vi "MsgLog.vi"(10 "OP_ID":refnum<vi>) -> ()   [LabVIEW 2019, in "MsgShowAndLog.lvlib"]
uses:
  MsgShowAndLog.lvlib
  Ctrl/MsgPageSelect.ctl
  Ctrl/MsgTyp.ctl
  Ctrl/MsgDataInput.ctl
  Ctrl/LogType.ctl
  <vilib>/Utility/miscctls.llb/LVPositionTypeDef.ctl
  global/MsgQue.vi
  Commonly VI.lvlib
panel:
  in  "OP":string
  in  "DataIn":T1={"MsgPageSelect"=enum."Action", "LogType"=enum."Manual", "Msg"="", "Time"=""}
  in  "Type":T4=enum."IO"
  in  "Enum":T2
  in  "error in":errorcluster
  in  "Main_msgTable":enum32{"系統訊息", "通訊訊息", "IO訊息", "動作訊息", "報警訊息"}(tab)
  in  "SystemMsg":i32(listbox)
  in  "RobotMsg":i32(listbox)
  in  "IOMsg":i32(listbox)
  in  "ActionMsg":i32(listbox)
  in  "AlarmMsg":i32(listbox)
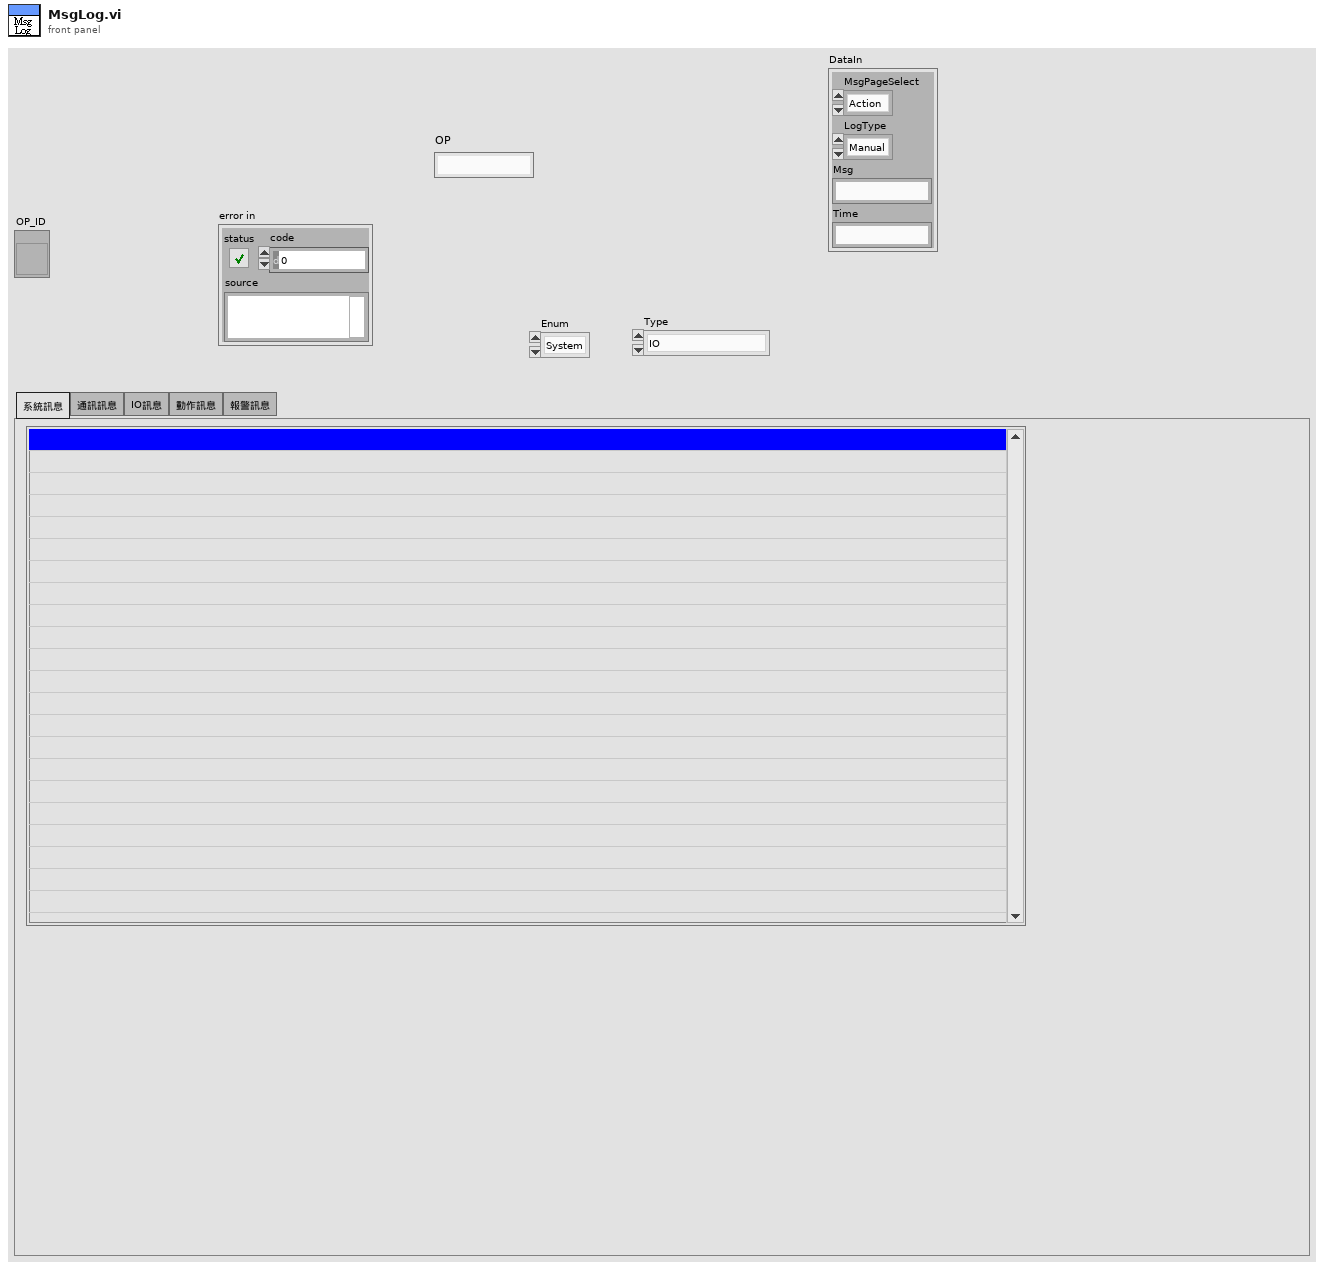
[diagram p1: front panel]
types:
  T1 = typedef "MsgDataInput.ctl" = cluster{"MsgPageSelect":T2, "LogType":T3, "Msg":string, "Time":string}
  T2 = typedef "MsgShowAndLog.lvlib/MsgPageSelect.ctl" = enum16{"System", "Comm", "IO", "Action", "Alarm"}
  T3 = typedef "MsgShowAndLog.lvlib/LogType.ctl" = enum16{"Auto", "Manual", "Handshake", "Error"}
  T4 = typedef "MsgShowAndLog.lvlib/MsgTyp.ctl" = enum16{"SYS", "COMM", "IO", "Action", "Alarm"}
  T5 = typedef "LVPositionTypeDef.ctl" = cluster{"Left":i32, "Top":i32}
  T6 = typedef "LVBoundsTypeDef.ctl" = cluster{"Width":u32, "Height":u32}
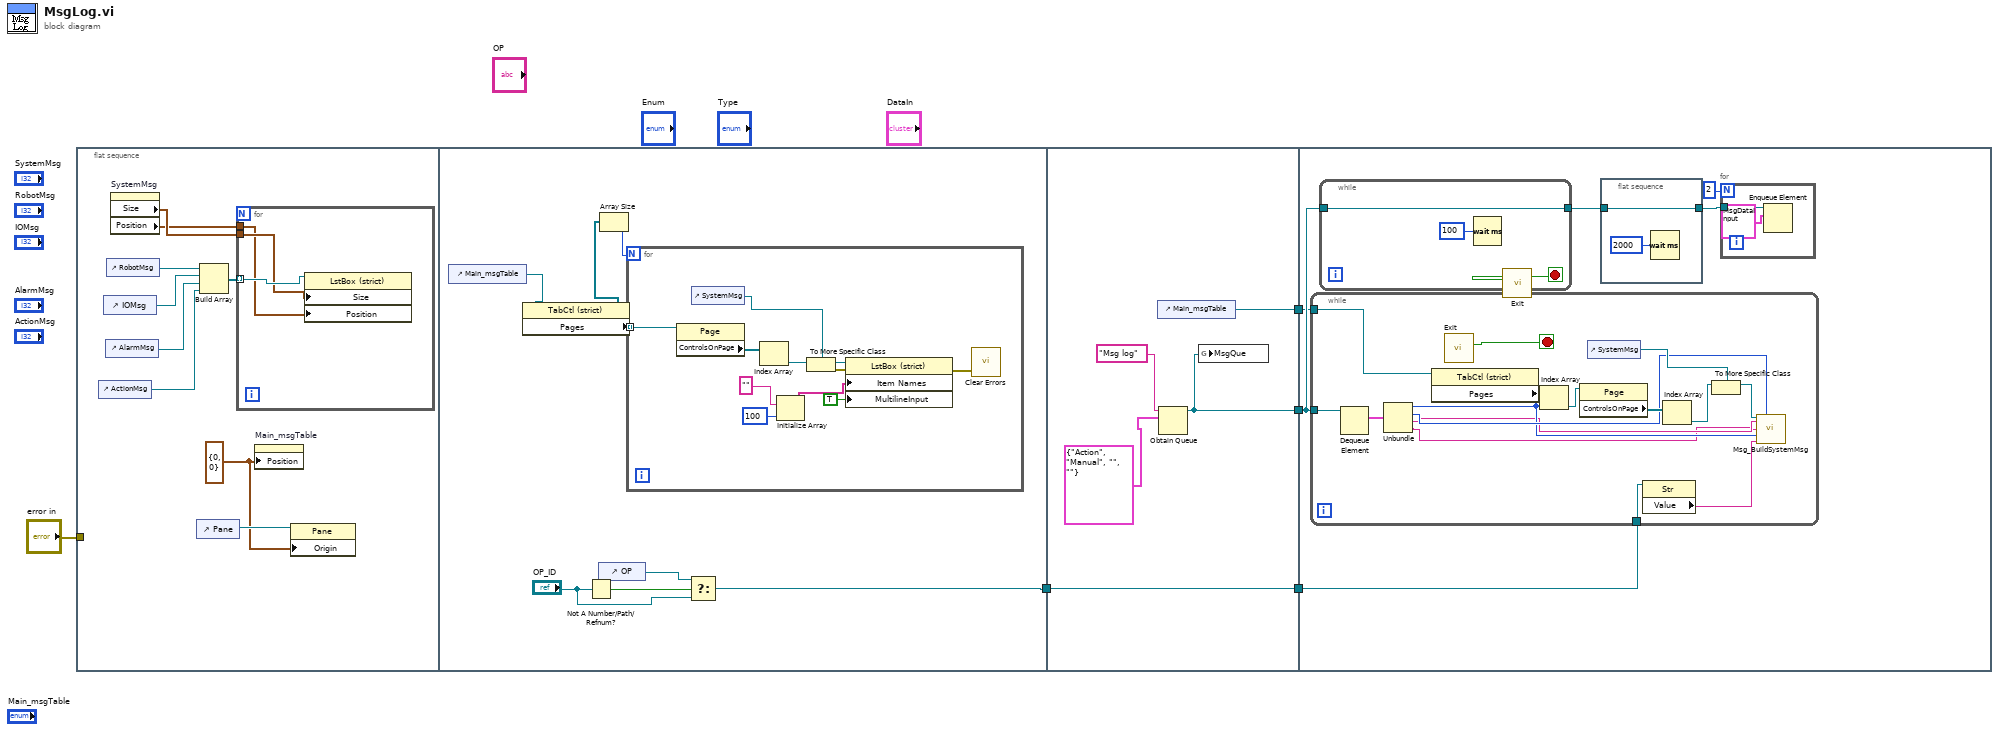
[diagram p0: block diagram]
diagram:
  n1 = flat-sequence {
    tunnel: "error in" -> [_]
    tunnel: [w20] -> w2
    tunnel: [w36] -> w5
    tunnel: [w39] -> w3
    tunnel: w2 -> [w39]
    tunnel: [w38] -> w1
    tunnel: w5 -> [w46]
    tunnel: w3 -> [w42]
    tunnel: w1 -> [w41]
    frame #0 {
      w6 = T5 {"Left"=0, "Top"=0} ("Position")
      n2 = control-ref of="ActionMsg"() -> (w11:refnum<vi>)
      n3 = control-ref of="IOMsg"() -> (w13:refnum<vi>)
      n4 = control-ref of="AlarmMsg"() -> (w12:refnum<vi>)
      n5 = control-ref of="RobotMsg"() -> (w14:refnum<vi>)
      n6 = property on="SystemMsg" class="LstBox (strict)"() -> ("Size"=w9:T6, "Position"=w8:T5)  [unwired: 2 in, 2 out]
      n7 = control-ref of="Pane"() -> (w7:refnum<vi>)
      n8 = Build Array(w14, w13, w12, w11) -> (w10:refnum<vi>[])
      n9 = for {
        tunnel: w10 -> [w17] mode=indexing
        tunnel: w9 -> [w16]
        tunnel: w8 -> [w15]
        n10 = property class="LstBox (strict)"(reference=w17, "Size"=w16, "Position"=w15) -> ()  [unwired: 1 in, 2 out]
      }
      n11 = property on="Main_msgTable" class="TabCtl (strict)"("Position"=w6) -> ()  [unwired: 2 in, 2 out]
      n12 = property class="Pane"(reference=w7, "Origin"=w6) -> ()  [unwired: 1 in, 2 out]
    }
    frame #1 {
      n13 = control-ref of="Main_msgTable"() -> (w18:refnum<vi>)
      n14 = property class="TabCtl (strict)"(reference=w18) -> ("Pages"=w24:refnum<vi>[])  [unwired: 1 in, 2 out]
      n15 = Not A Number/Path/Refnum?(number/path/refnum="OP_ID") -> (NaN/Path/Refnum?=w22:bool)
      n16 = control-ref of="OP"() -> (w19:refnum<vi>)
      n17 = Array Size(array=w24) -> (size(s)=w23:i32)
      n18 = for {
        N: w23 -> [_]
        tunnel: w24 -> [w35] mode=indexing
        n19 = property class="Page"(reference=w35) -> ("ControlsOnPage"=w34:refnum<vi>[])  [unwired: 1 in, 2 out]
        n20 = control-ref of="SystemMsg"() -> (w26:refnum<vi>)
        n21 = Index Array(array=w34) -> (element=w33:refnum<vi>)  [unwired: 1 in]
        n22 = Initialize Array("" ("name (unnamed)"), 100 ("dimension size")) -> (w30:string[])
        n23 = To More Specific Class(target class=w26, reference=w33) -> (specific class reference=w32:refnum<vi>, error out=w31:errorcluster)  [unwired: 1 in]
        n24 = property class="LstBox (strict)"(reference=w32, error in=w31, "Item Names"=w30, "MultilineInput"=TRUE ("Multiple Line Input")) -> (error out=w27:errorcluster)  [unwired: 1 out]
        n25 = call <vilib>:"Clear Errors.vi"("error in (no error)"=w27) -> ()  [unwired: 5 in, 2 out]
      }
      n26 = Select(t=w19, s=w22, f="OP_ID") -> (s? t:f=w20:refnum<vi>)
    }
    frame #2 {
      n27 = control-ref of="Main_msgTable"() -> (w38:refnum<vi>)
      n28 = Obtain Queue(name (unnamed)="Msg log", element data type=T1 {"MsgPageSelect"=enum."Action", "LogType"=enum."Manual", "Msg"="", "Time"=""} ("DataIn 2")) -> (queue out=w36:refnum<queue>)  [unwired: 3 in, 2 out]
      n29 = global write "MsgQue.vi" "MsgQue"(w36) -> ()
    }
    frame #3 {
      n30 = while {
        tunnel: w46 -> [w69]
        tunnel: w42 -> [w59]
        tunnel: w41 -> [w58]
        stop <- w62 stop-if-true
        n31 = Dequeue Element(queue=w69) -> (element=w68:T1)  [unwired: 2 in, 3 out]
        n32 = Unbundle(w68) -> ("MsgPageSelect"=w56:T2, "LogType"=w57:T3, "Msg"=w55:string, "Time"=w54:string)
        n33 = property class="TabCtl (strict)"(reference=w58) -> ("Pages"=w67:refnum<vi>[])  [unwired: 1 in, 2 out]
        n34 = call "Exit.vi"() -> ("ExitOut"=w62:bool)  [unwired: 11 in]
        n35 = Index Array(array=w67, index=w56) -> (element=w66:refnum<vi>)
        n36 = property class="Page"(reference=w66) -> ("ControlsOnPage"=w65:refnum<vi>[])  [unwired: 1 in, 2 out]
        n37 = control-ref of="SystemMsg"() -> (w61:refnum<vi>)
        n38 = property class="Str"(reference=w59) -> ("Value"=w63:string)  [unwired: 1 in, 2 out]
        n39 = Index Array(array=w65) -> (element=w64:refnum<vi>)  [unwired: 1 in]
        n40 = To More Specific Class(target class=w61, reference=w64) -> (specific class reference=w60:refnum<vi>)  [unwired: 1 in, 1 out]
        n41 = call "Msg_BuildSystemMsg.vi"("ListBoxRef"=w60, "LogType"=w57, "Data"=w55, "Time"=w54, "MsgPageSelect"=w56, "User"=w63) -> ()  [unwired: 10 in]
      }
      n42 = while {
        tunnel: w46 -> [w52]
        tunnel: [w52] -> w44
        stop <- w51 stop-if-true
        n43 = Wait (ms)(milliseconds to wait=u32 100) -> ()  [unwired: 1 out]
        n44 = call "Exit.vi"() -> ("ExitOut"=w51:bool)  [unwired: 11 in]
      }
      n45 = flat-sequence {
        tunnel: [w50] -> w45
        tunnel: w44 -> [w50]
        frame #0 {
          n46 = Wait (ms)(milliseconds to wait=u32 2000) -> ()  [unwired: 1 out]
        }
      }
      n47 = for {
        N: 2 -> [_]
        tunnel: w45 -> [w48]
        n48 = Enqueue Element(queue=w48, element=T1 {"MsgPageSelect"=enum."Action", "LogType"=enum."Manual", "Msg"="Exit", "Time"="Time"} ("DataIn 2")) -> ()  [unwired: 2 in, 3 out]
      }
    }
  }
